vi "set_aw_tune.vi"(6 "timeout (25000ms)":i32=25000, 7 "Power Mode or Target Power in W":string(combo), 8 "error in (no error)":errorcluster, 9 "Offset Power mW":i32, 10 "Index":i32 max=5 step=1, 11 "daemon reference in":refnum<k5>) -> (0 "error out":errorcluster, 2 "response":string, 3 "daemon reference out":refnum<k5>, 5 "command out":string="random")   [LabVIEW 2017]
doc: "<b>Command: </b>\"set_aw_tune\"\n\n<b>Description: </b> This command sets the airwatts delta power tuning parameter for the desired power mode or target power value in W (57-900)\n\n<b>Parameters: </b>index (0-5), power mode, offset power in mW\n____________________________________________\nDIPC 692 Daemon API 10.0.0.1\nSam Tee - Dyson Technology Ltd\nCopyright (c) 2024, Dyson Technology Ltd"
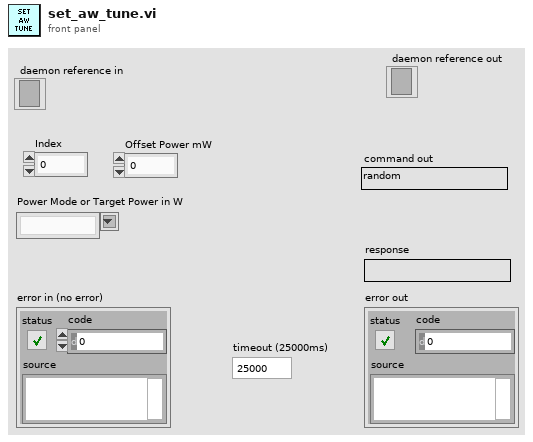
[diagram p1: front panel]
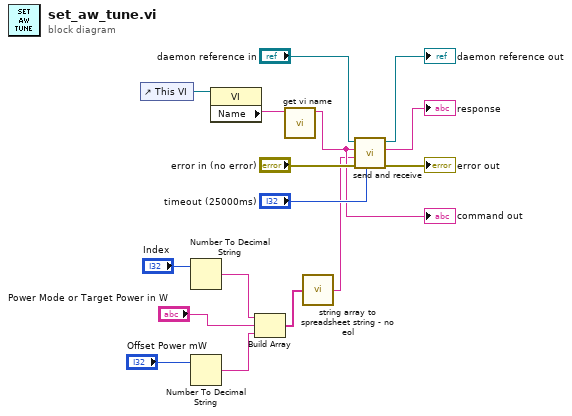
[diagram p0: block diagram]
diagram:
  n1 = control-ref of="This VI"() -> (w10:refnum<vi>)
  n2 = Number To Decimal String(number="Index") -> (decimal integer string=w4:string)  [unwired: 1 in]
  n3 = Number To Decimal String(number="Offset Power mW") -> (decimal integer string=w3:string)  [unwired: 1 in]
  n4 = property class="VI"(reference=w10) -> ("Name"=w9:string)  [unwired: 1 in, 2 out]
  n5 = Build Array(w4, "Power Mode or Target Power in W", w3) -> (w2:string[])
  n6 = call "get vi name.vi"("library.lvlib:name.vi"=w9) -> ("vi name"=w8:string)  [unwired: 10 in]
  "command out" <- w8
  n7 = call "string array to spreadsheet string - no eol.vi"("string array"=w2) -> ("spreadsheet string - no eol"=w7:string)
  n8 = call "send and receive.vi"("timeout (25000ms)"="timeout (25000ms)", "error in (no error)"="error in (no error)", "data"=w7, "command"=w8, "daemon reference in"="daemon reference in") -> ("error out"=→"error out":errorcluster, "response"=→"response":string, "daemon reference out"=→"daemon reference out":refnum<k5>)  [unwired: 4 in]
